vi "Teleop.vi"(10 "Match Info":T14={"Autonomous Elapsed Seconds"=0.0, "TeleOp Elapsed Seconds"=0.0, "Disabled Elapsed Seconds"=0.0, "Visited Autonomous"=FALSE, "Visited TeleOp"=FALSE, "Visited Disabled"=FALSE, "Autonomous Settings"={"Autonomous Style"=enum."Independent", "VI Refnum"=refnum}}, 11 "Call Context":T15) -> ()   [LabVIEW 2013]
doc: "This VI is called for each TeleOp packet received from the DS where the robot is not disabled. It is often used to read from the joysticks and update I/O or to update setpoints for timed control loops. It should complete and return within 20 milliseconds or it may miss DS packets."
uses:
  <vilib>/Rock Robotics/WPI/DriverStation/WPI_DriverStationDerivedRobotMode.ctl
  <vilib>/Rock Robotics/WPI/DriverStation/WPI_DriverStationMatch Info.ctl
  <vilib>/Rock Robotics/WPI/Solenoid/WPI_SolenoidDevRef.ctl
  <vilib>/Rock Robotics/SystemInterfaces/Typedef/FPGA_TypedefSolenoidModule.ctl
  <vilib>/Rock Robotics/WPI/Solenoid/WPI_SolenoidChannel.ctl
  <vilib>/Rock Robotics/WPI/RobotDrive/WPI_RobotDriveDevRef.ctl
  <vilib>/Rock Robotics/WPI/MotorControl/WPI_MotorControlDeviceRef.ctl
  <vilib>/Rock Robotics/SystemInterfaces/Typedef/FPGA_TypedefDigitalModule.ctl
  <vilib>/Rock Robotics/SystemInterfaces/DIO/FPGA_DIOPWMChannel.ctl
  <vilib>/Rock Robotics/WPI/PWM/WPI_PWMDeadband.ctl
  <vilib>/Rock Robotics/WPI/CAN/Jaguar/SubVIs/WPI_CANJaguar_ControlMode.ctl
  <vilib>/Rock Robotics/WPI/PWM/WPI_PWMTransform_ConPane.ctl
  <vilib>/Rock Robotics/WPI/Joystick/WPI_JoystickDevRef.ctl
  <vilib>/Rock Robotics/WPI/Joystick/WPI_JoystickDeviceEnum.ctl
  <vilib>/Rock Robotics/WPI/Solenoid/WPI_SolenoidValue.ctl
  Robot Global Data.vi
  <vilib>/Rock Robotics/WPI/Solenoid/WPI_SolenoidSetEnum.vi
  <vilib>/Rock Robotics/WPI/Joystick/WPI_JoystickGetSetRefNum.vi
  <vilib>/Rock Robotics/WPI/RobotDrive/WPI_RobotDriveGetSetRefNum.vi
panel:
  out "distance":dbl(slide)=125.0 scale=0.0..250.0 scale format="%3d"
  out "Waveform Chart 2":dbl(graph)
  out "Waveform Chart":dbl(graph)
  out "Robot_Heading_Debug":dbl(knob) scale=0.0..360.0
  out "iJoystick_1 2":T1
  out "iJoystick_1":T1
  out "iLeft_Right_Motor":T3={"DevStatus"={"status"=FALSE, "code"=0, "source"=""}, "Motors[]"=[], "Square Inputs"=FALSE, "Max Output"=1.0, "Isochronous"=FALSE}
  out "iLoad_CylinderI":T11={"DevStatus"={"status"=FALSE, "code"=0, "source"=""}, "Solenoid Module"=enum."Solenoid Module 1", "Forward Solenoid Channel"=enum."Invalid", "Reverse Solenoid Channel"=enum."Invalid"}
  out "iShooter_Cylinder":T11={"DevStatus"={"status"=FALSE, "code"=0, "source"=""}, "Solenoid Module"=enum."Solenoid Module 1", "Forward Solenoid Channel"=enum."Invalid", "Reverse Solenoid Channel"=enum."Invalid"}
  out "Numeric 1":dbl(slide) scale=0.0..100.0
  out "Boolean 2":bool
  out "Boolean 1":bool
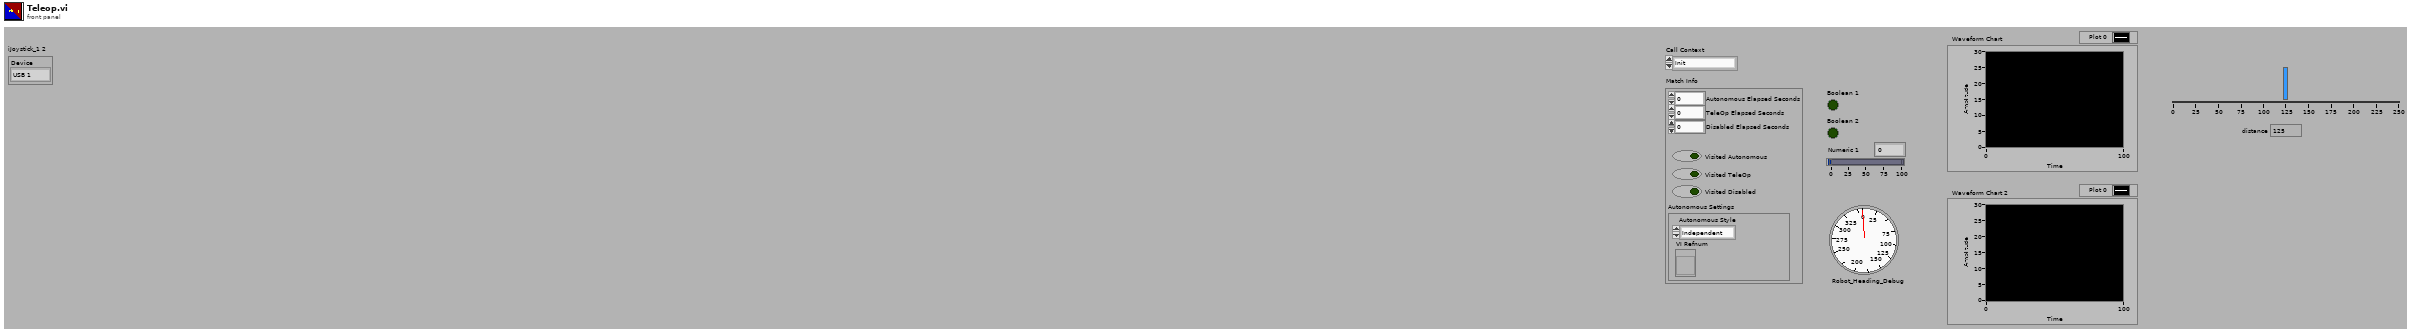
[diagram p1: front panel]
types:
  T1 = typedef "WPI_JoystickDevRef.ctl" = cluster{"Device":T2}
  T2 = typedef "WPI_JoystickDeviceEnum.ctl" = enum16{"USB 1", "USB 2", "USB 3", "USB 4", "Kinect 1", "Kinect 2"}
  T3 = typedef "WPI_RobotDriveDevRef.ctl" = cluster{"DevStatus":errorcluster, "Motors[]":T4[], "Square Inputs":bool, "Max Output":dbl, "Isochronous":bool}
  T4 = typedef "WPI_MotorControlDeviceRef.ctl" = cluster{"DeviceStatus":errorcluster, "Type":enum16{"PWM", "CAN"}, "PWM":cluster{"Digital Module":T5, "PWM Channel":T6, "DeadBand":T7}, "CAN":cluster{"Device Number":u8, "Control Mode":T8, "Semaphore":T9, "Max Vout":dbl}, "Invert":bool, "TransformRef":T10, "InvTransformRef":T10}
  T5 = typedef "FPGA_TypedefDigitalModule.ctl" = enum16{"Digital Module 1", "Digital Module 2"}
  T6 = typedef "FPGA_DIOPWMChannel.ctl" = enum8{"PWM 1", "PWM 2", "PWM 3", "PWM 4", "PWM 5", "PWM 6", "PWM 7", "PWM 8", "PWM 9", "PWM 10", "Invalid"}
  T7 = typedef "WPI_PWMDeadband.ctl" = cluster{"Name":string, "maxPositivePwm":i32, "minPositivePwm":i32, "centerPwm":i32, "maxNegativePwm":i32, "minNegativePwm":i32, "angularRange":u16}
  T8 = typedef "WPI_CANJaguar_ControlMode.ctl" = enum8{"Percent VBus", "Current", "Speed", "Position", "Voltage"}
  T9 = typedef "Semaphore RefNum" = refnum<k1>
  T10 = typedef "WPI_PWMTransform_ConPane.ctl" = refnum<vi>
  T11 = typedef "WPI_SolenoidDevRef.ctl" = cluster{"DevStatus":errorcluster, "Solenoid Module":T12, "Forward Solenoid Channel":T13, "Reverse Solenoid Channel":T13}
  T12 = typedef "FPGA_TypedefSolenoidModule.ctl" = enum16{"Solenoid Module 1", "Solenoid Module 2"}
  T13 = typedef "WPI_SolenoidChannel.ctl" = enum8{"Solenoid 1", "Solenoid 2", "Solenoid 3", "Solenoid 4", "Solenoid 5", "Solenoid 6", "Solenoid 7", "Solenoid 8", "Invalid"}
  T14 = typedef "WPI_DriverStationMatch Info.ctl" = cluster{"Autonomous Elapsed Seconds":dbl, "TeleOp Elapsed Seconds":dbl, "Disabled Elapsed Seconds":dbl, "Visited Autonomous":bool, "Visited TeleOp":bool, "Visited Disabled":bool, "Autonomous Settings":cluster{"Autonomous Style":enum16{"Iterative", "Independent"}, "VI Refnum":refnum<vi>}}
  T15 = typedef "WPI_DriverStationDerivedRobotMode.ctl" = enum16{"Init", "Execute", "Stop"}
  T16 = typedef "WPI_JoystickButtonState.ctl" = cluster{"Button 1":bool, "Button 2":bool, "Button 3":bool, "Button 4":bool, "Button 5":bool, "Button 6":bool, "Button 7":bool, "Button 8":bool, "Button 9":bool, "Button 10":bool, "Button 11":bool, "Button 12":bool}
  T17 = cluster{"axis 1 (x)":dbl, "axis 2 (y)":dbl, "axis 3 (throttle)":dbl, "axis 4":dbl, "axis 5":dbl, "axis 6":dbl}
  T18 = typedef "WPI_SolenoidValue.ctl" = enum16{"Off", "On", "Forward", "Reverse"}
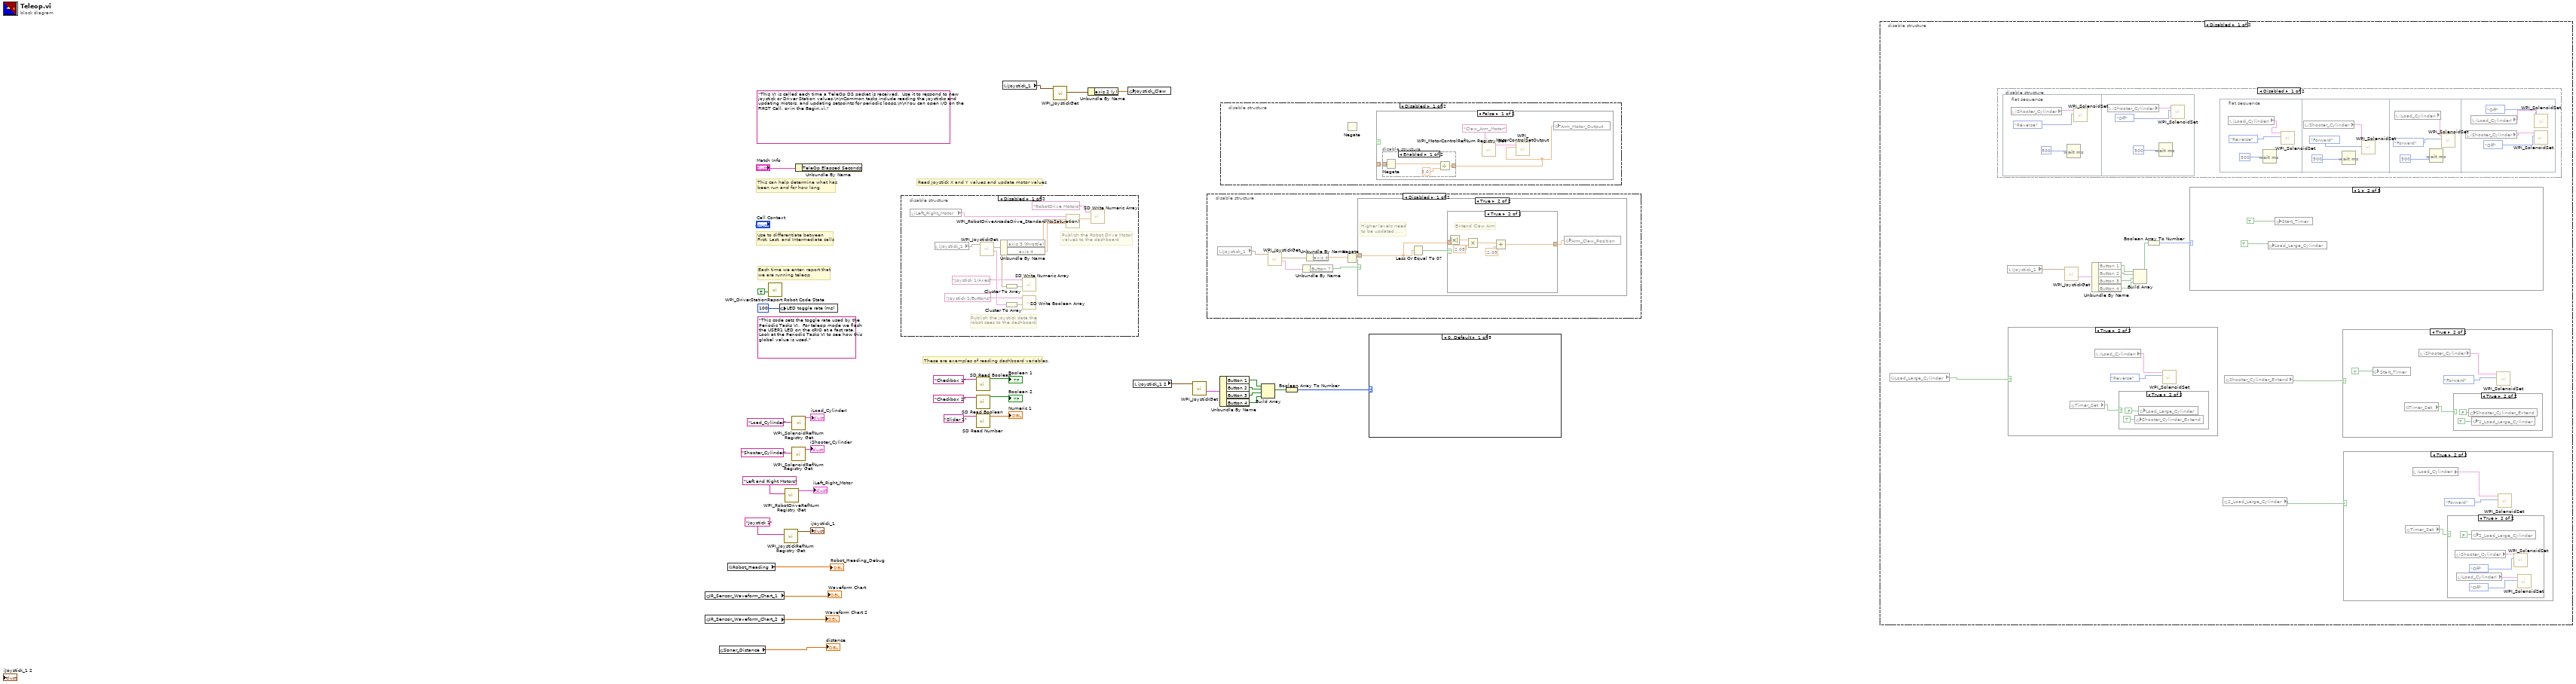
[diagram p0: block diagram]
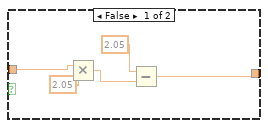
[diagram p7: hidden frame]
diagram:
  (unwired) "This code sets the toggle rate used by the Periodic Tasks VI.  For teleop mode we flash the USER1 LED on the cRIO at a fast rate.  Look at the Periodic Tasks VI to see how this global value is used."
  (unwired) "This VI is called each time a TeleOp DS packet is received.  Use it to respond to new joystick or Driver Station values.\n\nCommon tasks include reading the joysticks and updating motors, and updating setpoints for periodic loops.\n\nYou can open I/O on the FIRST Call, or in the Begin.vi."
  # "These are examples of reading dashboard variables."
  # "Each time we enter, report that\nwe are running teleop"
  # "Use to differentiate between\nFirst, Last, and Intermediate calls"
  # "This can help determine what has\nbeen run and for how long"
  # "Read Joystick X and Y values and update motor values"
  n1 = global read "Robot Global Data.vi" "IR_Sensor_Waveform_Chart_1"() -> (→"Waveform Chart":dbl)
  n2 = global read "Robot Global Data.vi" "IR_Sensor_Waveform_Chart_2"() -> (→"Waveform Chart 2":dbl)
  n3 = global read "Robot Global Data.vi" "Sonar_Distance"() -> (→"distance":dbl)
  n4 = global read "Robot Global Data.vi" "Robot_Heading"() -> (→"Robot_Heading_Debug":dbl)
  n5 = call <vilib>:"WPI_DriverStationReport Robot Code State.vi"("TeleOp"=TRUE ("Autonomous")) -> ()  [unwired: 10 in, 1 out]
  n6 = global write "Robot Global Data.vi" "LED toggle rate (ms)"(u32 100 ("LED ms toggle rate")) -> ()
  n7 = call <vilib>:"WPI_JoystickRefNum Registry Get.vi"("refnum name"="Joystick 1") -> ("JoystickDevRef"=→"iJoystick_1":T1)  [unwired: 1 in, 9 out]
  n8 = call <vilib>:"WPI_RobotDriveRefNum Registry Get.vi"("refnum name"="Left and Right Motors") -> ("RobotDriveDevRef"=→"iLeft_Right_Motor":T3)  [unwired: 1 in, 9 out]
  n9 = call <vilib>:"WPI_SolenoidRefNum Registry Get.vi"("refnum name"="Shooter_Cylinder") -> ("SolenoidDevRef"=→"iShooter_Cylinder":T11)  [unwired: 9 in, 1 out]
  n10 = call <vilib>:"WPI_SolenoidRefNum Registry Get.vi"("refnum name"="Load_Cylinder") -> ("SolenoidDevRef"=→"iLoad_CylinderI":T11)  [unwired: 9 in, 1 out]
  n11 = Unbundle By Name("Match Info") -> ()  [unwired: 1 out]
  n12 = disable-structure shown="Disabled" {
    frame Disabled {
      # "Publish the Robot Drive Motor\nvalues to the dashboard"
      # "Publish the joystick data the\nrobot sees to the dashboard"
      n13 = local read "iLeft_Right_Motor"() -> (w34:T3)
      n14 = local read "iJoystick_1"() -> (w33:T1)
      n15 = call <vilib>:"WPI_JoystickGet.vi"("JoystickDevRef"=w33) -> ("Buttons"=w42:T16, "Axes"=w39:T17)  [unwired: 1 in, 4 out]
      n16 = Unbundle By Name(w39) -> ("axis 3 (throttle)"=w44:dbl, "axis 4"=w43:dbl)
      n17 = Cluster To Array(cluster=w39) -> (array=w38:dbl[])
      n18 = Cluster To Array(cluster=w42) -> (array=w41:bool[])
      n19 = call <vilib>:"SD Write Numeric Array.vi"("Numeric Array"=w38, "Name"="Joystick 1/Axes") -> ()  [unwired: 8 in, 2 out]
      n20 = call <vilib>:"SD Write Boolean Array.vi"("Boolean Array"=w41, "Name"="Joystick 1/Buttons") -> ()  [unwired: 8 in, 2 out]
      n21 = call <vilib>:"WPI_RobotDriveArcadeDrive_Standard(NoSaturation).vi"("Y axis value"=w43, "X axis value"=w44, "RobotDriveDevRef"=w34) -> ("Motor Values"=w35:dbl[])  [unwired: 1 in, 7 out]
      n22 = call <vilib>:"SD Write Numeric Array.vi"("Numeric Array"=w35, "Name"="RobotDrive Motors") -> ()  [unwired: 8 in, 2 out]
    }
    frame Enabled {
    }
  }
  n23 = call <vilib>:"SD Read Boolean.vi"("Name"="Checkbox 1" ("refnum name")) -> ("Boolean"=→"Boolean 1":bool)  [unwired: 8 in, 2 out]
  n24 = call <vilib>:"SD Read Boolean.vi"("Name"="Checkbox 2" ("refnum name")) -> ("Boolean"=→"Boolean 2":bool)  [unwired: 8 in, 2 out]
  n25 = call <vilib>:"SD Read Number.vi"("Name"="Slider 1" ("refnum name")) -> ("Numeric"=→"Numeric 1":dbl)  [unwired: 8 in, 2 out]
  n26 = local read "iJoystick_1"() -> (w3:T1)
  n27 = call <vilib>:"WPI_JoystickGet.vi"("JoystickDevRef"=w3) -> ("Axes"=w2:T17)  [unwired: 1 in, 5 out]
  n28 = Unbundle By Name(w2) -> ("axis 2 (y)"=w1:dbl)
  n29 = global write "Robot Global Data.vi" "Joystick_Claw"(w1) -> ()
  n30 = local read "iJoystick_1 2"() -> (w15:T1)
  n31 = call <vilib>:"WPI_JoystickGet.vi"("JoystickDevRef"=w15) -> ("Buttons"=w14:T16)  [unwired: 1 in, 5 out]
  n32 = disable-structure shown="Disabled" {
    frame Disabled {
      n33 = local read "iJoystick_1"() -> (w50:T1)
      n34 = call <vilib>:"WPI_JoystickGet.vi"("JoystickDevRef"=w50) -> ("Buttons"=w46:T16, "Axes"=w49:T17)  [unwired: 1 in, 4 out]
      n35 = Unbundle By Name(w46) -> ("Button 7"=w45:bool)
      n36 = Unbundle By Name(w49) -> ("axis 4"=w48:dbl)
      n37 = Negate(x=w48) -> (-x=w47:dbl)
      n38 = case shown="True" w45 {
        tunnel: w47 -> [_ w51]
        frame False {
        }
        frame True {
          # "Higher levels need \nto be updated . . ."
          n39 = Less Or Equal To 0?(x=w51) -> (x <= 0?=w53:bool)
          n40 = case shown="True" w53 {
            tunnel: w51 -> [w57 w64]
            tunnel: [w54 w59] -> w52
            frame False {
              n41 = Multiply(x=w57, y=2.05) -> (x*y=w55:dbl)
              n42 = Subtract(x=2.05, y=w55) -> (x-y=w54:dbl)
            }
            frame True {
              # "Extend Claw Arm"
              n43 = Absolute Value(x=w64) -> (abs(x)=w63:dbl)
              n44 = Multiply(x=w63, y=2.05) -> (x*y=w61:dbl)
              n45 = Add(x=w61, y=2.05) -> (x+y=w59:dbl)
            }
          }
          n46 = global write "Robot Global Data.vi" "Arm_Claw_Position"(w52) -> ()
        }
      }
    }
    frame Enabled {
    }
  }
  n47 = Unbundle By Name(w14) -> ("Button 1"=w12:bool, "Button 2"=w11:bool, "Button 3"=w10:bool, "Button 4"=w9:bool)
  n48 = disable-structure shown="Disabled" {
    frame Disabled {
      n49 = Negate() -> (x=w65:dbl, -x=w66:dbl)
      n50 = case shown="False" w67 {
        tunnel: _ -> [w68 _]
        frame False {
          n51 = disable-structure shown="Enabled" {
            disable-tunnel: w68 -> [w73 _]
            disable-tunnel: [w72 _] -> w69
            frame Enabled {
              n52 = Negate(x=w73) -> (-x=w74:dbl)
              n53 = Divide(x=w74, y=3.0) -> (x/y=w72:dbl)
            }
            frame Disabled {
            }
          }
          n54 = call <vilib>:"WPI_MotorControlRefNum Registry Get.vi"("refnum name"="Claw_Arm_Motor") -> ("MotorControlDevRef"=w70:T4)  [unwired: 1 in, 9 out]
          n55 = call <vilib>:"WPI_MotorControlSetOutput.vi"("Output"=w69, "MotorControlDevRef"=w70) -> ()  [unwired: 3 in, 7 out]
          n56 = global write "Robot Global Data.vi" "Arm_Motor_Output"(w69) -> ()
        }
        frame True {
        }
      }
    }
    frame Enabled {
    }
  }
  n57 = Build Array(w12, w11, w10, w9) -> (w8:bool[])
  n58 = Boolean Array To Number(Boolean array=w8) -> (number=w13:u32)
  n59 = case shown="0, Default" w13 {
    frame 0, Default {
    }
    frame 1 {
      # "Button 1"
      n60 = flat-sequence {
        frame #0 {
          n61 = local read "iLoad_CylinderI"() -> (w78:T11)
          n62 = Wait (ms)(milliseconds to wait=20) -> ()  [unwired: 1 out]
          n63 = call-poly <vilib>:"WPI_SolenoidSet.vi"("Value"=WPI_SolenoidValue."Reverse", "SolenoidDevRef"=w78) -> ()  [unwired: 8 in, 2 out]
        }
        frame #1 {
          n64 = local read "iLoad_CylinderI"() -> (w79:T11)
          n65 = call-poly <vilib>:"WPI_SolenoidSet.vi"("Value"=WPI_SolenoidValue."Off", "SolenoidDevRef"=w79) -> ()  [unwired: 8 in, 2 out]
        }
      }
    }
    frame 2 {
      # "Button 2"
      n66 = flat-sequence {
        frame #0 {
          n67 = local read "iShooter_Cylinder"() -> (w83:T11)
          n68 = Wait (ms)(milliseconds to wait=20) -> ()  [unwired: 1 out]
          n69 = call-poly <vilib>:"WPI_SolenoidSet.vi"("Value"=WPI_SolenoidValue."Forward", "SolenoidDevRef"=w83) -> ()  [unwired: 8 in, 2 out]
        }
        frame #1 {
          n70 = local read "iShooter_Cylinder"() -> (w84:T11)
          n71 = call-poly <vilib>:"WPI_SolenoidSet.vi"("Value"=WPI_SolenoidValue."Off", "SolenoidDevRef"=w84) -> ()  [unwired: 8 in, 2 out]
        }
      }
    }
    frame 4 {
      n72 = flat-sequence {
        frame #0 {
          # "Button 3"
          n73 = local read "iLoad_CylinderI"() -> (w88:T11)
          n74 = Wait (ms)(milliseconds to wait=100) -> ()  [unwired: 1 out]
          n75 = call-poly <vilib>:"WPI_SolenoidSet.vi"("Value"=WPI_SolenoidValue."Forward", "SolenoidDevRef"=w88) -> ()  [unwired: 8 in, 2 out]
        }
        frame #1 {
          n76 = local read "iLoad_CylinderI"() -> (w89:T11)
          n77 = call-poly <vilib>:"WPI_SolenoidSet.vi"("Value"=WPI_SolenoidValue."Off", "SolenoidDevRef"=w89) -> ()  [unwired: 8 in, 2 out]
        }
      }
    }
    frame 8 {
      n78 = flat-sequence {
        frame #0 {
          # "Button 4"
          n79 = local read "iShooter_Cylinder"() -> (w93:T11)
          n80 = Wait (ms)(milliseconds to wait=20) -> ()  [unwired: 1 out]
          n81 = call-poly <vilib>:"WPI_SolenoidSet.vi"("Value"=WPI_SolenoidValue."Reverse", "SolenoidDevRef"=w93) -> ()  [unwired: 8 in, 2 out]
        }
        frame #1 {
          n82 = local read "iShooter_Cylinder"() -> (w94:T11)
          n83 = call-poly <vilib>:"WPI_SolenoidSet.vi"("Value"=WPI_SolenoidValue."Off", "SolenoidDevRef"=w94) -> ()  [unwired: 8 in, 2 out]
        }
      }
    }
  }
  n84 = disable-structure shown="Disabled" {
    frame Disabled {
      n85 = global read "Robot Global Data.vi" "Load_Large_Cylinder"() -> (w98:bool)
      n86 = disable-structure shown="Disabled" {
        frame Disabled {
          n87 = flat-sequence {
            frame #0 {
              n88 = local read "iShooter_Cylinder"() -> (w122:T11)
              n89 = Wait (ms)(milliseconds to wait=500) -> ()  [unwired: 1 out]
              n90 = call-poly <vilib>:"WPI_SolenoidSet.vi"("Value"=WPI_SolenoidValue."Reverse", "SolenoidDevRef"=w122) -> ()  [unwired: 1 in, 9 out]
            }
            frame #1 {
              n91 = local read "iShooter_Cylinder"() -> (w125:T11)
              n92 = Wait (ms)(milliseconds to wait=500) -> ()  [unwired: 1 out]
              n93 = call-poly <vilib>:"WPI_SolenoidSet.vi"("Value"=WPI_SolenoidValue."Off", "SolenoidDevRef"=w125) -> ()  [unwired: 1 in, 9 out]
            }
          }
          n94 = flat-sequence {
            frame #0 {
              n95 = local read "iLoad_CylinderI"() -> (w109:T11)
              n96 = Wait (ms)(milliseconds to wait=500) -> ()  [unwired: 1 out]
              n97 = call-poly <vilib>:"WPI_SolenoidSet.vi"("Value"=WPI_SolenoidValue."Reverse", "SolenoidDevRef"=w109) -> ()  [unwired: 8 in, 2 out]
            }
            frame #1 {
              n98 = local read "iShooter_Cylinder"() -> (w112:T11)
              n99 = Wait (ms)(milliseconds to wait=500) -> ()  [unwired: 1 out]
              n100 = call-poly <vilib>:"WPI_SolenoidSet.vi"("Value"=WPI_SolenoidValue."Forward", "SolenoidDevRef"=w112) -> ()  [unwired: 8 in, 2 out]
            }
            frame #2 {
              n101 = local read "iLoad_CylinderI"() -> (w115:T11)
              n102 = Wait (ms)(milliseconds to wait=500) -> ()  [unwired: 1 out]
              n103 = call-poly <vilib>:"WPI_SolenoidSet.vi"("Value"=WPI_SolenoidValue."Forward", "SolenoidDevRef"=w115) -> ()  [unwired: 8 in, 2 out]
            }
            frame #3 {
              n104 = local read "iShooter_Cylinder"() -> (w119:T11)
              n105 = local read "iLoad_CylinderI"() -> (w118:T11)
              n106 = call-poly <vilib>:"WPI_SolenoidSet.vi"("Value"=WPI_SolenoidValue."Off", "SolenoidDevRef"=w119) -> ()  [unwired: 8 in, 2 out]
              n107 = call-poly <vilib>:"WPI_SolenoidSet.vi"("Value"=WPI_SolenoidValue."Off", "SolenoidDevRef"=w118) -> ()  [unwired: 8 in, 2 out]
            }
          }
        }
        frame Enabled {
        }
      }
      n108 = local read "iJoystick_1"() -> (w106:T1)
      n109 = case shown="True" w98 {
        frame False {
        }
        frame True {
          n110 = global read "Robot Global Data.vi" "Timer_Set"() -> (w140:bool)
          n111 = local read "iLoad_CylinderI"() -> (w142:T11)
          n112 = case shown="True" w140 {
            frame False {
            }
            frame True {
              n113 = global write "Robot Global Data.vi" "Shooter_Cylinder_Extend"(TRUE) -> ()
              n114 = global write "Robot Global Data.vi" "Load_Large_Cylinder"(FALSE) -> ()
            }
          }
          n115 = call-poly <vilib>:"WPI_SolenoidSet.vi"("Value"=WPI_SolenoidValue."Reverse", "SolenoidDevRef"=w142) -> ()  [unwired: 8 in, 2 out]
        }
      }
      n116 = call <vilib>:"WPI_JoystickGet.vi"("JoystickDevRef"=w106) -> ("Buttons"=w105:T16)  [unwired: 1 in, 5 out]
      n117 = Unbundle By Name(w105) -> ("Button 1"=w103:bool, "Button 2"=w102:bool, "Button 3"=w101:bool, "Button 4"=w100:bool)
      n118 = Build Array(w103, w102, w101, w100) -> (w99:bool[])
      n119 = Boolean Array To Number(Boolean array=w99) -> (number=w104:u32)
      n120 = case shown="1" w104 {
        frame 0, Default {
        }
        frame 1 {
          n121 = global write "Robot Global Data.vi" "Load_Large_Cylinder"(TRUE) -> ()
          n122 = global write "Robot Global Data.vi" "Start_Timer"(TRUE) -> ()
        }
        frame 2 {
        }
        frame 4 {
        }
        frame 8 {
        }
      }
      n123 = global read "Robot Global Data.vi" "2_Load_Large_Cylinder"() -> (w96:bool)
      n124 = global read "Robot Global Data.vi" "Shooter_Cylinder_Extend"() -> (w97:bool)
      n125 = case shown="True" w97 {
        frame False {
        }
        frame True {
          n126 = global write "Robot Global Data.vi" "Start_Timer"(TRUE) -> ()
          n127 = global read "Robot Global Data.vi" "Timer_Set"() -> (w136:bool)
          n128 = local read "iShooter_Cylinder"() -> (w135:T11)
          n129 = case shown="True" w136 {
            frame False {
            }
            frame True {
              n130 = global write "Robot Global Data.vi" "Shooter_Cylinder_Extend"(FALSE) -> ()
              n131 = global write "Robot Global Data.vi" "2_Load_Large_Cylinder"(TRUE) -> ()
            }
          }
          n132 = call-poly <vilib>:"WPI_SolenoidSet.vi"("Value"=WPI_SolenoidValue."Forward", "SolenoidDevRef"=w135) -> ()  [unwired: 8 in, 2 out]
        }
      }
      n133 = case shown="True" w96 {
        frame False {
        }
        frame True {
          n134 = global read "Robot Global Data.vi" "Timer_Set"() -> (w127:bool)
          n135 = local read "iLoad_CylinderI"() -> (w126:T11)
          n136 = case shown="True" w127 {
            frame False {
            }
            frame True {
              n137 = local read "iShooter_Cylinder"() -> (w132:T11)
              n138 = local read "iLoad_CylinderI"() -> (w131:T11)
              n139 = global write "Robot Global Data.vi" "2_Load_Large_Cylinder"(FALSE) -> ()
              n140 = call-poly <vilib>:"WPI_SolenoidSet.vi"("Value"=WPI_SolenoidValue."Off", "SolenoidDevRef"=w132) -> ()  [unwired: 8 in, 2 out]
              n141 = call-poly <vilib>:"WPI_SolenoidSet.vi"("Value"=WPI_SolenoidValue."Off", "SolenoidDevRef"=w131) -> ()  [unwired: 8 in, 2 out]
            }
          }
          n142 = call-poly <vilib>:"WPI_SolenoidSet.vi"("Value"=WPI_SolenoidValue."Forward", "SolenoidDevRef"=w126) -> ()  [unwired: 8 in, 2 out]
        }
      }
    }
    frame Enabled {
    }
  }
